vi "Add Device.vi"(8 "Error In":errorcluster, 10 "Device UID":string, 11 "IP Connection":refnum<class "IP Connection.lvclass">) -> (0 "Error Out":errorcluster, 3 "Ambient Light Bricklet":refnum<class "Temperature IR Bricklet.lvclass">)   [LabVIEW 2011, in "Tinkerforge.lvlib" / "Temperature IR Bricklet.lvclass"]
doc: "This VI adds an Temperature IR Bricklet to the stack."
uses:
  Temperature IR Bricklet.lvclass
  IP Connection/IP Connection.lvclass
  Device/Device.lvclass
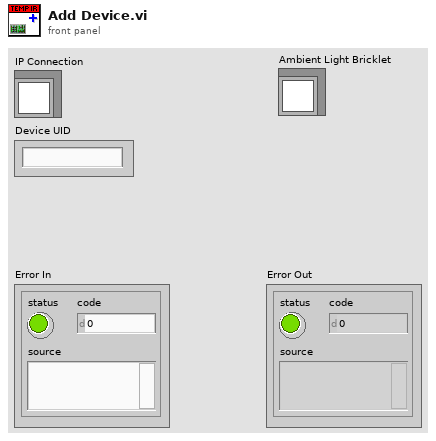
[diagram p1: front panel]
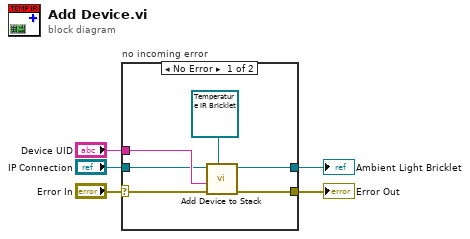
[diagram p0: block diagram]
diagram:
  n1 = case "no incoming error" shown="No Error" "Error In" {
    selector: "Error In" -> [w9 w12]
    tunnel: [w6 w12] -> w4
    tunnel: "IP Connection" -> [w8 _]
    tunnel: "Device UID" -> [w10 _]
    tunnel: [w7 _] -> w1
    frame No Error {
      n2 = call "Add Device to Stack.vi"("Device in"=refnum<class "Temperature IR Bricklet.lvclass"> refnum ("Tinkerforge.lvlib:Ambient Light Bricklet.lvclass"), "error in (no error)"=w9, "Device UID"=w10, "IP Connection in"=w8) -> ("error out"=w6:errorcluster, "Device out"=w7:refnum<class "Temperature IR Bricklet.lvclass">)  [unwired: 6 in]
    }
    frame Error {
    }
  }
  "Error Out" <- w4
  "Ambient Light Bricklet" <- w1
